vi "Attach Arduino Shield.vi"(8 "error in (no error)":errorcluster, 10 "Arduino Shield":refnum<class "Arduino Shield.lvclass">, 11 "Arduino in":refnum<class "Arduino.lvclass">) -> (0 "error out":errorcluster, 3 "Arduino out":refnum<class "Arduino.lvclass">)   [LabVIEW 2020, in "Arduino.lvclass"]
uses:
  Arduino.lvclass
  Interfaces/Arduino Shield/Arduino Shield.lvclass
  Arduino.lvclass/Arduino.ctl
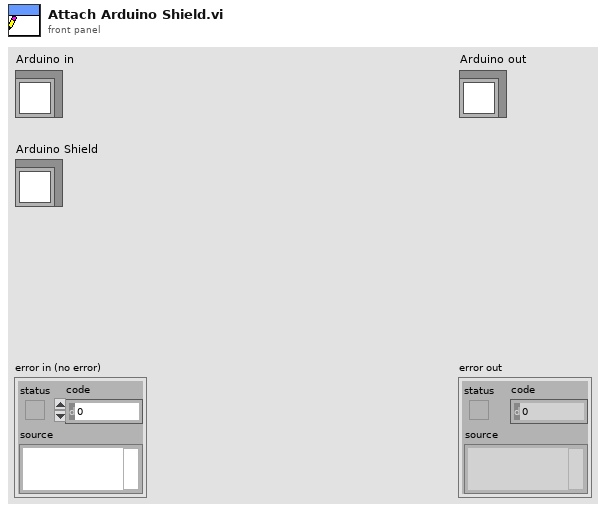
[diagram p1: front panel]
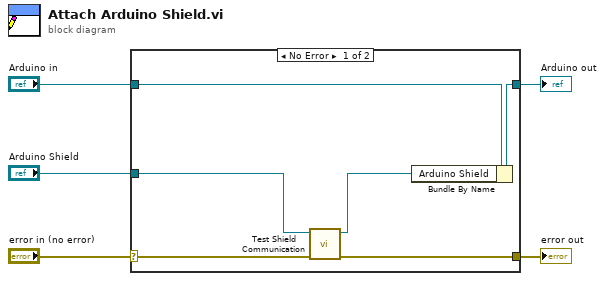
[diagram p0: block diagram]
diagram:
  n1 = case shown="No Error" "error in (no error)" {
    selector: "error in (no error)" -> [w11 w12]
    tunnel: [w8 w12] -> w4
    tunnel: [w9 w13] -> w2
    tunnel: "Arduino in" -> [w10 w13]
    tunnel: "Arduino Shield" -> [w7 _]
    frame No Error {
      n2 = call-dynamic "Test Shield Communication.vi"("error in (no error)"=w11, "Arduino Shield in"=w7) -> ("error out"=w8:errorcluster, "Arduino Shield out"=w6:refnum<class "Arduino Shield.lvclass">)  [unwired: 8 in]
      n3 = Bundle By Name(cluster=w10, "Arduino Shield"=w6) -> (w9:refnum<class "Arduino.lvclass">)
    }
    frame Error {
    }
  }
  "error out" <- w4
  "Arduino out" <- w2
